vi "Part 1.vi"(11 "Input":string) -> (3 "Output":i64)   [LabVIEW 2021]
uses:
  <userlib>/_OpenG.lib/string/string.llb/Convert EOLs (String)__ogtk.vi
panel:
  out "Intensity Graph":i16[][](graph)
  out "Start":cluster{"Row":i32, "Col":i32}
  out "End":cluster{"Row":i32, "Col":i32}
  out "Grid":string[][](array[string])
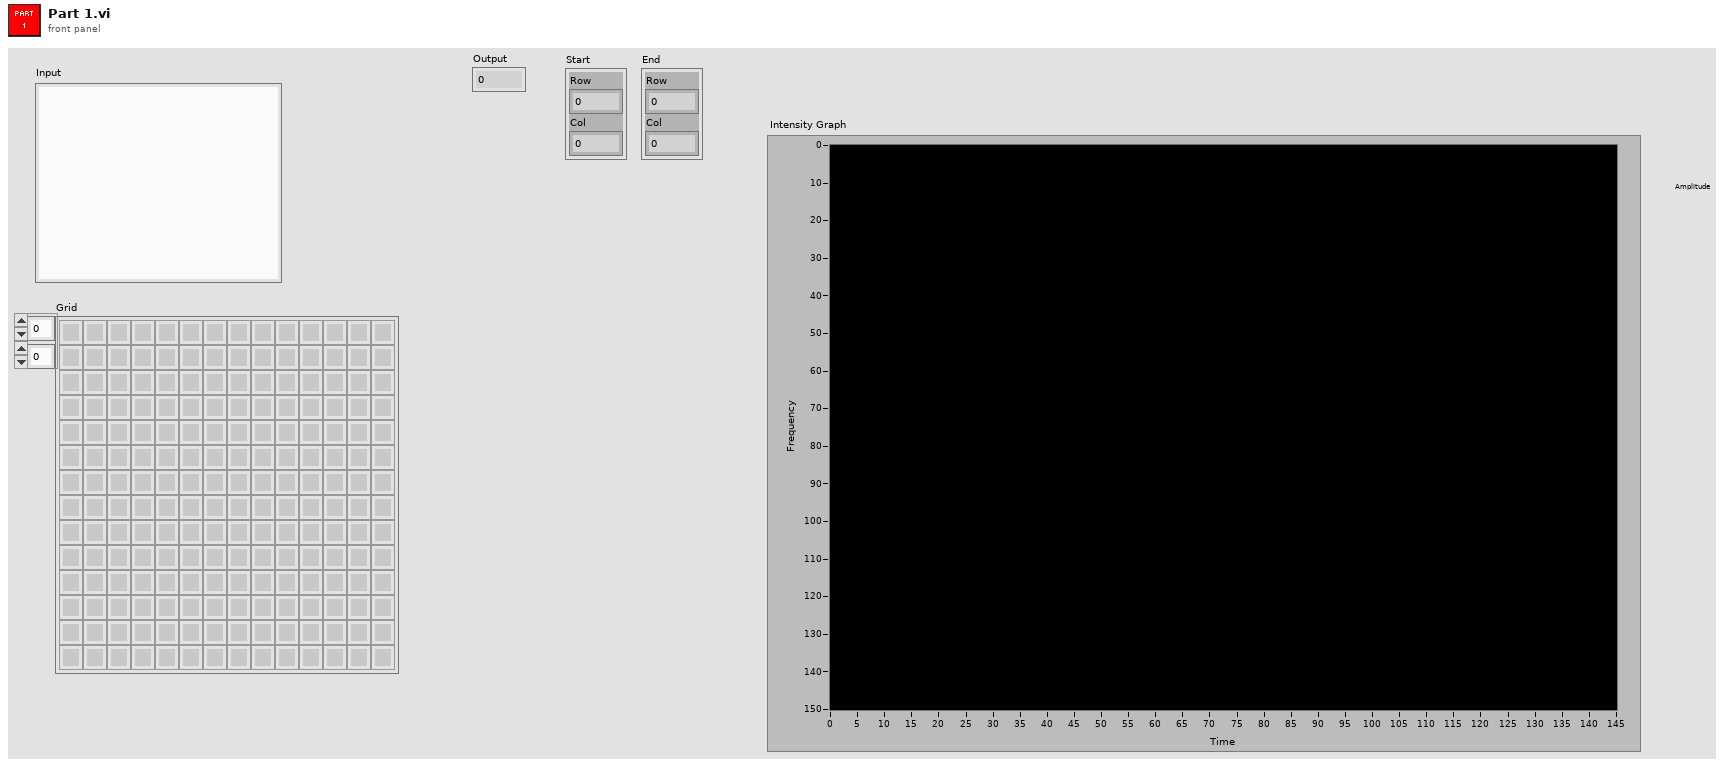
[diagram p1: front panel]
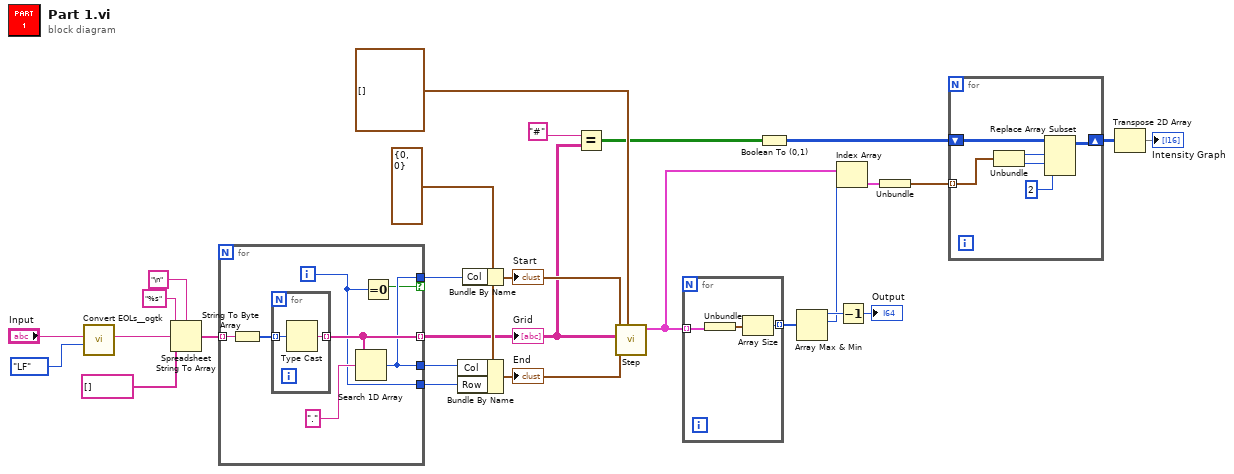
[diagram p0: block diagram]
diagram:
  w19 = cluster{"Row":i32, "Col":i32} {"Row"=0, "Col"=0}
  n1 = call-poly <userlib>:"Convert EOLs__ogtk.vi"("Convert to:"=enum16{"CR", "LF", "CRLF"}."LF", "String in"="Input") -> ("String out"=w23:string)  [unwired: 9 in]
  n2 = Spreadsheet String To Array(delimiter (Tab)="\n", format string="%s", spreadsheet string=w23, array type (2D Dbl)=string[] []) -> (array=w21:string[])
  n3 = for {
    tunnel: w21 -> [w34] mode=indexing
    tunnel: [w32] -> w7 mode=indexing
    tunnel: [w30] -> w18
    tunnel: [w30] -> w20 if=w29
    tunnel: [w28] -> w17
    i -> [w28]
    n4 = String To Byte Array(string=w34) -> (unsigned byte array=w33:u8[])
    n5 = for {
      tunnel: w33 -> [w36] mode=indexing
      tunnel: [w35] -> w32 mode=indexing
      n6 = Type Cast(x=w36) -> (*(type *) &x=w35:string)  [unwired: 1 in]
    }
    n7 = Search 1D Array(1D array=w32, element=".") -> (index of element=w30:i32)  [unwired: 1 in]
    n8 = Equal To 0?(x=w28) -> (x = 0?=w29:bool)
  }
  "Grid" <- w7
  n9 = Bundle By Name(cluster=w19, "Col"=w18, "Row"=w17) -> (w16:cluster{"Row":i32, "Col":i32})
  "End" <- w16
  n10 = Bundle By Name(cluster=w19, "Col"=w20) -> (w15:cluster{"Row":i32, "Col":i32})
  "Start" <- w15
  n11 = Equal?(x="#", y=w7) -> (x = y?=w4:bool[][])
  n12 = call "Step.vi"("Path In"=cluster{"Row":i32, "Col":i32}[] [], "End"=w16, "Grid"=w7, "Current Pos"=w15) -> ("Paths Out"=w8:cluster{cluster{"Row":i32, "Col":i32}[]}[])  [unwired: 7 in]
  n13 = for {
    tunnel: w8 -> [w39] mode=indexing
    tunnel: [w37] -> w13 mode=indexing
    n14 = Unbundle(w39) -> (w38:cluster{"Row":i32, "Col":i32}[])
    n15 = Array Size(array=w38) -> (size(s)=w37:i32)
  }
  n16 = Boolean To (0,1)(Boolean=w4) -> (0, 1=w3:i16[][])
  n17 = Array Max & Min(array=w13) -> (max value=w12:i32, max index (indices)=w10:i32)  [unwired: 2 out]
  n18 = Index Array(array=w8, index=w10) -> (element=w9:cluster{cluster{"Row":i32, "Col":i32}[]})
  n19 = Decrement(x=w12) -> (x-1=→"Output":i32)
  n20 = Unbundle(w9) -> (w5:cluster{"Row":i32, "Col":i32}[])
  n21 = for {
    tunnel: w5 -> [w44] mode=indexing
    shift-right: [w40] -> w2
    shift-left: w3 -> [w45]
    n22 = Unbundle(w44) -> ("Row"=w43:i32, "Col"=w42:i32)
    n23 = Replace Array Subset(array=w45, new element=2, index (row)=w43, index (col)=w42) -> (w40:i16[][])
  }
  n24 = Transpose 2D Array(2D array=w2) -> (transposed array=→"Intensity Graph":i16[][])
